vi "3P_Chrg.vi"(0 "Parallel Task in":refnum<k21>, 1 "Capacity (Ah)":dbl format="%#.6g", 2 "C rate Setpoint":dbl format="%#.6g", 3 "Charge Voltage Setpoint":dbl format="%#.6g", 5 "P task error in":errorcluster, 9 "NHR VISA in":refnum<visa-resource-name>, 11 "NHR error in":errorcluster caption="NHR error in (no error)", 12 "ChargeCyclePath":path=path "C:/Users/ga11/Desktop/VI/results/3PtestCharge.lvm" caption="Filename", 13 "Current Cutoff":dbl) -> (4 "parallel task out":refnum<k21>, 6 "parallel task error out":errorcluster, 10 "VISA resource name out":refnum<visa-resource-name>, 15 "NHR error out":errorcluster)   [LabVIEW 2020]
uses:
  <vilib>/DAQmx/read.llb/DAQmx Read (Analog 1D DBL NChan 1Samp).vi
  <vilib>/DAQmx/miscellaneous.llb/DAQmx Fill In Error Info.vi
  <instrlib>/NH Research Regenerative Test Series/Public/Data/Read (Ave Current).vi
  <instrlib>/NH Research Regenerative Test Series/Public/Data/Low Level/Fetch (Ave Voltage).vi
  <instrlib>/NH Research Regenerative Test Series/Public/Data/Low Level/Fetch (Ave True Power).vi
  <instrlib>/NH Research Regenerative Test Series/NH Research Regenerative Test Series.lvlib
panel:
  out "Ave Current (A)":dbl
  out "Ave Voltage (V)":dbl
  out "Ave True Power (W)":dbl
  out "Status Byte Register":T1
  out "Current Compare":dbl
  out "Battery1ChargeCurrent":dbl
  out "Battery2chargeCurrent":dbl
  out "Battery3chargeCurrent":dbl
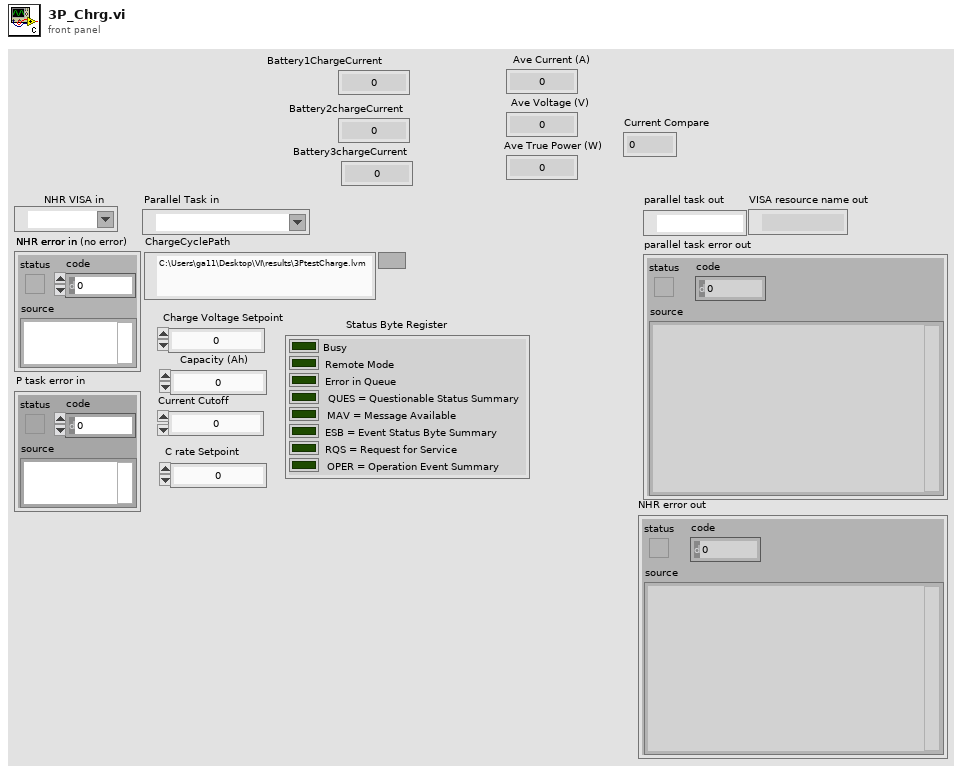
[diagram p1: front panel]
types:
  T1 = cluster{"Busy":bool, "Remote Mode":bool, "Error in Queue":bool, "QUES = Questionable Status Summary":bool, "MAV = Message Available":bool, "ESB = Event Status Byte Summary":bool, "RQS = Request for Service":bool, "OPER = Operation Event Summary":bool}
  T2 = cluster{"Voltage Enabled":bool, "Current Enabled":bool, "Power Enabled":bool, "Resistance Enabled":bool}
  T3 = cluster{"data[0]":dbl, "data[1]":dbl, "data[2]":dbl, "data[3]":dbl, "data[4]":dbl, "data[5]":dbl, "data[6]":dbl, "data[7]":dbl, "data[8]":dbl, "data[9]":dbl}
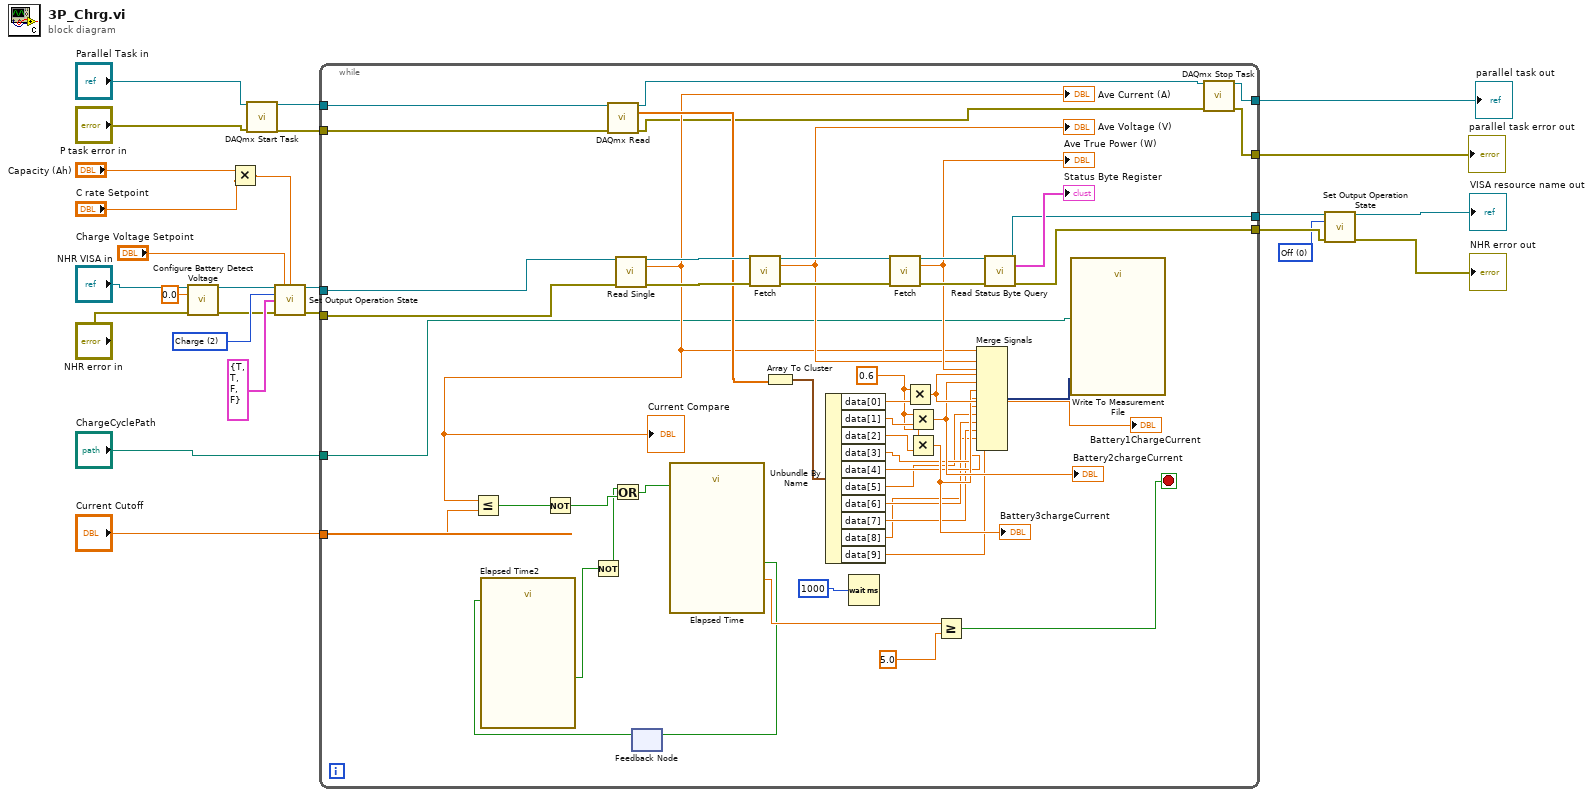
[diagram p0: block diagram]
diagram:
  w10 = 0 items=["Off", "Standby", "Charge", "Discharge", "Battery"] ("Mode (0: Off)")
  w18 = 2 items=["Off", "Standby", "Charge", "Discharge", "Battery"] ("Mode (0: Off)")
  n1 = call <instrlib>:"Configure Battery Detect Voltage.vi"("VISA resource name"="NHR VISA in", "Battery Detect Voltage (0V)"=0.0, "error in (no error)"="NHR error in") -> ("VISA resource name out"=w7:refnum<visa-resource-name>, "error out"=w6:errorcluster)  [unwired: 11 in]
  n2 = Multiply(x="Capacity (Ah)", y="C rate Setpoint") -> (x*y=w21:dbl)
  n3 = call <vilib>:"DAQmx Start Task.vi"("task/channels in"="Parallel Task in", "error in"="P task error in") -> ("task out"=w16:refnum<k21>, "error out"=w15:errorcluster)  [unwired: 12 in]
  n4 = call <vilib>:"Set Output Operation State.vi"("VISA resource name"=w7, "Voltage Setpoint (0 V)"="Charge Voltage Setpoint", "Current Setpoint (0 A)"=w21, "Mode (0: Off)"=w18, "Enable"=T2 {"Voltage Enabled"=TRUE, "Current Enabled"=TRUE, "Power Enabled"=FALSE, "Resistance Enabled"=FALSE}, "error in (no error)"=w6) -> ("VISA resource name out"=w25:refnum<visa-resource-name>, "error out"=w24:errorcluster)  [unwired: 8 in]
  n5 = while {
    tunnel: w25 -> [w70]
    tunnel: w24 -> [w69]
    tunnel: [w67] -> w12
    tunnel: [w66] -> w11
    tunnel: "Current Cutoff" -> [w61]
    tunnel: w15 -> [w33]
    tunnel: w16 -> [w32]
    tunnel: "ChargeCyclePath" -> [w31]
    tunnel: [w28] -> w2
    tunnel: [w27] -> w1
    stop <- w36 stop-if-true
    w51 = 0.6
    n6 = call-poly <vilib>:"DAQmx Read.vi"("task/channels in"=w32, "error in"=w33) -> ("task out"=w30:refnum<k21>, "data"=w64:dbl[], "error out"=w29:errorcluster)  [unwired: 11 in]
    n7 = call-poly <instrlib>:"Read Single.vi"("VISA resource name"=w70, "error in (no error)"=w69) -> ("VISA resource name out"=w75:refnum<visa-resource-name>, "Ave Current (A)"=w59:dbl, "error out"=w76:errorcluster)  [unwired: 11 in]
    "Ave Current (A)" <- w59
    "Current Compare" <- w59
    n8 = Less Or Equal?(x=w59, y=w61) -> (x <= y?=w50:bool)
    n9 = Not(x=w50) -> (.not. x?=w42:bool)
    n10 = feedback #1() -> (w34:bool)  [unwired: 1 in]
    n11 = call "Elapsed Time2"("Reset"=w34) -> ("Time has Elapsed"=w41:bool)  [unwired: 11 in, 7 out]
    n12 = Not(x=w41) -> (.not. x?=w40:bool)
    n13 = Or(x=w40, y=w42) -> (x .or. y?=w39:bool)
    n14 = call "Elapsed Time"("Reset"=w39) -> ("Elapsed Time (s)"=w38:dbl, "Time has Elapsed"=w35:bool)  [unwired: 11 in, 6 out]
    n15 = feedback-in #1(w35) -> ()
    n16 = call-poly <instrlib>:"Fetch.vi"("VISA resource name"=w75, "error in (no error)"=w76) -> ("VISA resource name out"=w74:refnum<visa-resource-name>, "Ave Voltage (V)"=w60:dbl, "error out"=w73:errorcluster)  [unwired: 11 in]
    "Ave Voltage (V)" <- w60
    n17 = Array To Cluster(array=w64) -> (cluster=w63:T3)
    n18 = Unbundle By Name(w63) -> ("data[0]"=w57:dbl, "data[1]"=w55:dbl, "data[2]"=w52:dbl, "data[3]"=w49:dbl, "data[4]"=w48:dbl, "data[5]"=w47:dbl, "data[6]"=w46:dbl, "data[7]"=w45:dbl, "data[8]"=w44:dbl, "data[9]"=w43:dbl)
    n19 = Wait (ms)(milliseconds to wait=1000) -> ()  [unwired: 1 out]
    n20 = call-poly <instrlib>:"Fetch.vi"("VISA resource name"=w74, "error in (no error)"=w73) -> ("VISA resource name out"=w72:refnum<visa-resource-name>, "Ave True Power (W)"=w65:dbl, "error out"=w71:errorcluster)  [unwired: 11 in]
    "Ave True Power (W)" <- w65
    n21 = Multiply(x=w51, y=w57) -> (x*y=w56:dbl)
    "Battery1ChargeCurrent" <- w56
    n22 = Multiply(x=w51, y=w55) -> (x*y=w54:dbl)
    "Battery2chargeCurrent" <- w54
    n23 = Multiply(x=w51, y=w52) -> (x*y=w53:dbl)
    "Battery3chargeCurrent" <- w53
    n24 = Greater Or Equal?(x=w38, y=5.0) -> (x >= y?=w36:bool)
    n25 = Merge Signals "Merge Signals"(w59, w60, w65, w56, w54, w53, w49, w48, w47, w46, w45, w44, w43) -> (w62:dynamicdata)
    n26 = call <instrlib>:"Read Status Byte Query.vi"("VISA resource name"=w72, "error in (no error)"=w71) -> ("VISA resource name out"=w67:refnum<visa-resource-name>, "Status Byte Register"=→"Status Byte Register":T1, "error out"=w66:errorcluster)  [unwired: 11 in]
    n27 = call "Write To Measurement File"("Signals"=w62, "Filename"=w31) -> ()  [unwired: 15 in, 3 out]
    n28 = call <vilib>:"DAQmx Stop Task.vi"("task/channels in"=w30, "error in"=w29) -> ("task out"=w28:refnum<k21>, "error out"=w27:errorcluster)  [unwired: 12 in]
  }
  "parallel task out" <- w2
  "parallel task error out" <- w1
  n29 = call <vilib>:"Set Output Operation State.vi"("VISA resource name"=w12, "Mode (0: Off)"=w10, "error in (no error)"=w11) -> ("VISA resource name out"=→"VISA resource name out":refnum<visa-resource-name>, "error out"=→"NHR error out":errorcluster)  [unwired: 11 in]
